vi "Get Wheel Separation.vi"(8 "error in (no error)":errorcluster, 11 "differential steering frame in":refnum<class "NI_Robotics_Differential Steering Frame.lvclass">) -> (0 "error out":errorcluster, 2 "wheel separation":dbl, 3 "differential steering frame out":refnum<class "NI_Robotics_Differential Steering Frame.lvclass">)   [LabVIEW 2017, in "NI_Robotics_Differential Steering Frame.lvclass"]
uses:
  <vilib>/robotics/Steering/Differential Steering Frame/NI_Robotics_Differential Steering Frame.lvclass
  <vilib>/robotics/Steering/Differential Steering Frame/NI_Robotics_Differential Steering Frame.lvclass/NI_Robotics_Differential Steering Frame.ctl
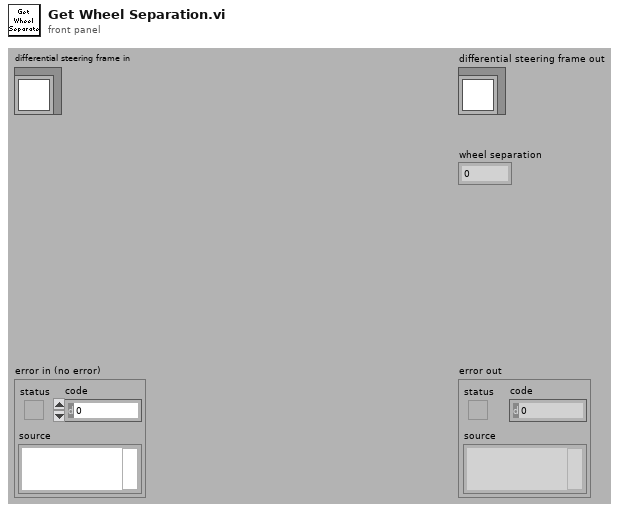
[diagram p1: front panel]
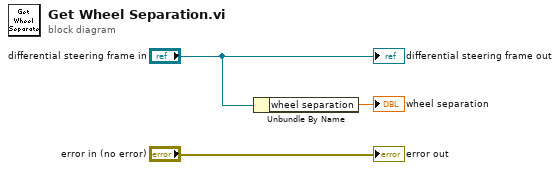
[diagram p0: block diagram]
diagram:
  n1 = Unbundle By Name("differential steering frame in") -> ("wheel separation"=→"wheel separation":dbl)
  "error out" <- "error in (no error)"
  "differential steering frame out" <- "differential steering frame in"
